vi "Write Timestamp Rule.vi"(8 "error in (no error)":errorcluster, 10 "Timestamp Rule":refnum<class "Timestamp Rule Interface.lvclass">, 11 "Timestamp Column in":refnum<class "Timestamp Column.lvclass">) -> (0 "error out":errorcluster, 3 "Timestamp Column out":refnum<class "Timestamp Column.lvclass">)   [LabVIEW 2020, in "Basic Columns.lvlib" / "Timestamp Column.lvclass"]
uses:
  Timestamp Column.lvclass
  Column Interface/Timestamp Rule Interface/Timestamp Rule Interface.lvclass
  Timestamp Column.lvclass/Timestamp Column.ctl
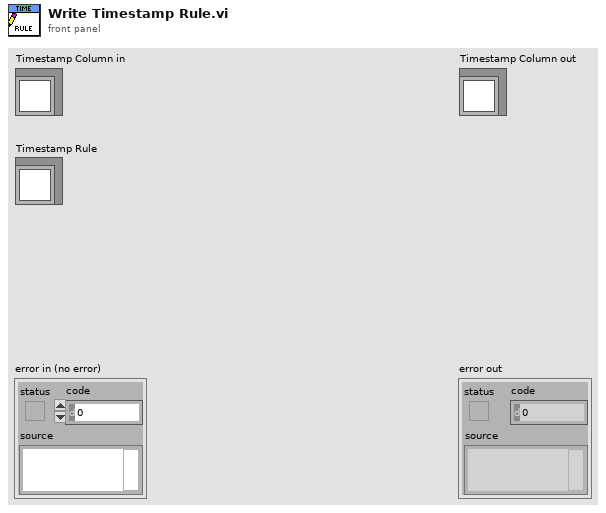
[diagram p1: front panel]
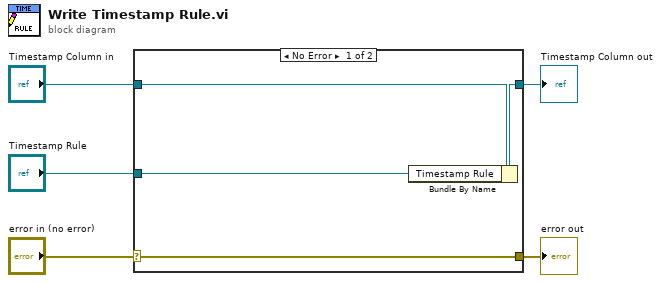
[diagram p0: block diagram]
diagram:
  n1 = case shown="No Error" "error in (no error)" {
    selector: "error in (no error)" -> [w9 w10]
    tunnel: [w9 w10] -> w4
    tunnel: [w7 w11] -> w2
    tunnel: "Timestamp Column in" -> [w8 w11]
    tunnel: "Timestamp Rule" -> [w6 _]
    frame No Error {
      n2 = Bundle By Name(cluster=w8, "Timestamp Rule"=w6) -> (w7:refnum<class "Timestamp Column.lvclass">)
    }
    frame Error {
    }
  }
  "error out" <- w4
  "Timestamp Column out" <- w2
